vi "Line Search Prep.vi"(5 "result":dbl[][](array[numeric]) format="%.2f", 6 "list of variables":i32[](array[numeric])=[0, 0], 7 "table":i32[][][](array[numeric]), 8 "TOLX":dbl=1e-07 format="%.2e", 9 "P":dbl[](array[numeric]) format="%.2f", 10 "X":dbl[](array[numeric]) format="%.2f", 11 "J":dbl[][](array[numeric]) format="%.2f") -> (0 "F(X)*F(X)":dbl format="%.2f", 1 "tolerance":dbl format="%.2f", 3 "X * Y":dbl format="%.2f")   [LabVIEW 2017, in "NI_Gmath.lvlib"]
uses:
  NI_Gmath.lvlib
  A x Vector.vi
  Real Dot Product.vi
  NI_AALBase.lvlib
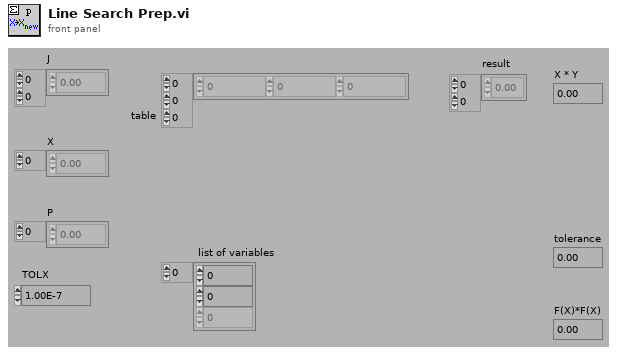
[diagram p1: front panel]
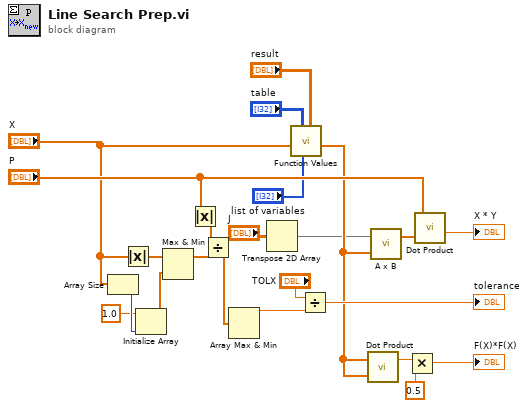
[diagram p0: block diagram]
diagram:
  n1 = Array Size(array="X") -> (size(s)=w8:i32)
  n2 = Absolute Value(x="X") -> (abs(x)=w10:dbl[])
  n3 = Initialize Array(1.0, w8) -> (w9:dbl[])
  n4 = Max & Min(x=w10, y=w9) -> (max(x,y)=w12:dbl[])  [unwired: 1 out]
  n5 = Absolute Value(x="P") -> (abs(x)=w11:dbl[])
  n6 = Divide(x=w11, y=w12) -> (x/y=w13:dbl[])
  n7 = Array Max & Min(array=w13) -> (max value=w15:dbl)  [unwired: 3 out]
  n8 = Transpose 2D Array(2D array="J") -> (transposed array=w5:dbl[][])
  n9 = call "Function Values.vi"("result"="result", "list of variables"="list of variables", "table"="table", "X"="X") -> ("F(X)"=w16:dbl[])  [unwired: 7 in]
  n10 = Divide(x="TOLX", y=w15) -> (x/y=→"tolerance":dbl)
  n11 = call-poly "Dot Product.vi"("Y Vector"=w16, "X Vector"=w16) -> ("X * Y"=w17:dbl)  [unwired: 1 out]
  n12 = call-poly "A x B.vi"("Vector"=w16, "A"=w5) -> ("A x Vector"=w6:dbl[])  [unwired: 1 out]
  n13 = Multiply(x=w17, y=0.5) -> (x*y=→"F(X)*F(X)":dbl)
  n14 = call-poly "Dot Product.vi"("Y Vector"=w6, "X Vector"="P") -> ("X * Y"=→"X * Y":dbl)  [unwired: 1 out]
